vi "Delacor_lib_QMH_Create Message Queue.vi"(8 "error in":errorcluster) -> (0 "error out":errorcluster, 3 "Message Queue":refnum<class "JQMH_Message Queue.lvclass">)   [LabVIEW 2024, in "JQMH_Message Queue.lvclass"]
doc: "This VI creates and initializes the message queue for a QMH Module. \nIf the message needs to be different for the given module, then create a child class of Message Queue and override the appropriate methods.\n____\nDQMH Framework: Palette 7.1.0.1503\nCopyright (c) 2025, DQMH Consortium"
uses:
  JQMH_Message Queue.lvclass
  Delacor_lib_QMH_Message--cluster.ctl
  JQMH_Message Queue.lvclass/JQMH_Message Queue.ctl
  Delacor_lib_QMH_Enqueue Message (Single).vi
  Delacor_lib_QMH_Set Message Queue.vi
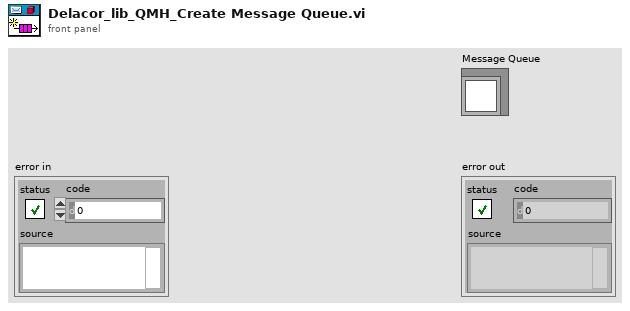
[diagram p1: front panel]
types:
  T1 = typedef "JQMH_Message Queue.lvclass/Delacor_lib_QMH_Message--cluster.ctl" = cluster{"Message":string, "Message Data":variant}
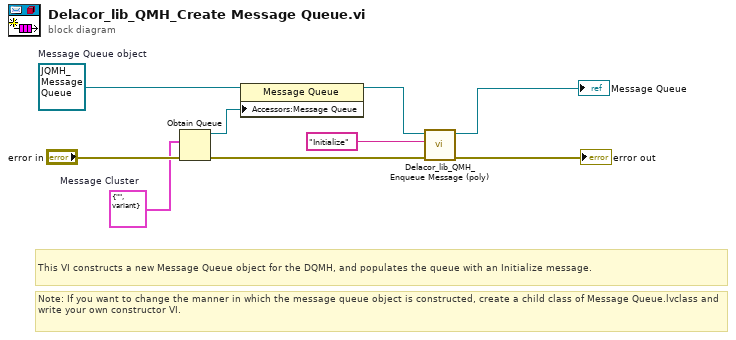
[diagram p0: block diagram]
diagram:
  w2 = T1 {"Message"="", "Message Data"=variant}  # Message Cluster
  w5 = refnum<class "JQMH_Message Queue.lvclass"> refnum  # Message Queue object
  # "Note: If you want to change the manner in which the message queue object is constructed, create a child class of Message Queue.lvclass and write your own constructor VI."
  # "This VI constructs a new Message Queue object for the DQMH, and populates the queue with an Initialize message."
  n1 = Obtain Queue(element data type=w2, error in (no error)="error in") -> (queue out=w1:refnum<queue>, error out=w7:errorcluster)  [unwired: 3 in, 1 out]
  n2 = property class="Message Queue"(reference=w5, "Accessors:Message Queue"=w1) -> (reference out=w3:refnum<class "JQMH_Message Queue.lvclass">)  [unwired: 1 in, 1 out]
  n3 = call-poly "Delacor_lib_QMH_Enqueue Message (poly).vi"("error in"=w7, "Message"="Initialize", "Message Queue in"=w3) -> ("error out"=→"error out":errorcluster, "Message Queue out"=→"Message Queue":refnum<class "JQMH_Message Queue.lvclass">)  [unwired: 7 in]
